vi "TDC_addHistogram.vi"(8 "Error In":errorcluster, 9 "Add":bool, 10 "Stop Channel":i32, 11 "Start Channel":i32) -> (0 "Error Out":errorcluster)   [LabVIEW 2011]
uses:
  tdcbase.dll
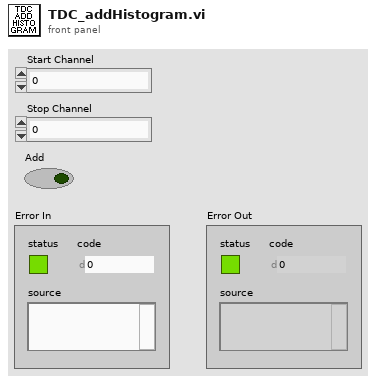
[diagram p1: front panel]
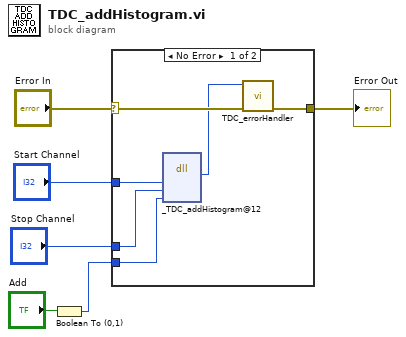
[diagram p0: block diagram]
diagram:
  n1 = Boolean To (0,1)(Boolean="Add") -> (0, 1=w1:i16)
  n2 = case shown="No Error" "Error In" {
    selector: "Error In" -> [w12 w13]
    tunnel: [w11 w13] -> w5
    tunnel: "Start Channel" -> [w9 _]
    tunnel: "Stop Channel" -> [w8 _]
    tunnel: w1 -> [w7 _]
    frame No Error {
      n3 = dll-call lib="X:/tdcbase.dll" fn="_TDC_addHistogram@12"("startChannel"=w9, "stopChannel"=w8, "add"=w7) -> ("return type"=w10:i32)  [unwired: 6 in, 2 out]
      n4 = call "TDC_errorHandler.vi"("Error In"=w12, "TDC Return Code"=w10) -> ("Error Out"=w11:errorcluster)  [unwired: 9 in]
    }
    frame Error {
    }
  }
  "Error Out" <- w5
